vi "camera test.vi"() -> ()   [LabVIEW 2023]
uses:
  <vilib>/DAQmx/create/channels.llb/DAQmx Create Channel (DO-Digital Output).vi
  <vilib>/DAQmx/configure/timing.llb/DAQmx Timing (Sample Clock).vi
  <vilib>/Analysis/NI_AALBase.lvlib
  <vilib>/DAQmx/write.llb/DAQmx Write (Digital 1D U32 1Chan NSamp).vi
panel:
  in  "task in":refnum<k21>
  in  "low time":dbl=0.01 format="%.6f"
  in  "high time":dbl=0.01 format="%.6f"
  in  "OK Button":bool
  out "Pulse Pattern":dbl[](array[numeric])
  in  "source":tag
  in  "lines 2":tag
  in  "lines":tag
  in  "Advanced Genicam::Command Timeout":u32=100 max=0
  in  "Stop (F)":bool
  out "Image Out 2":T1(plugin-control)
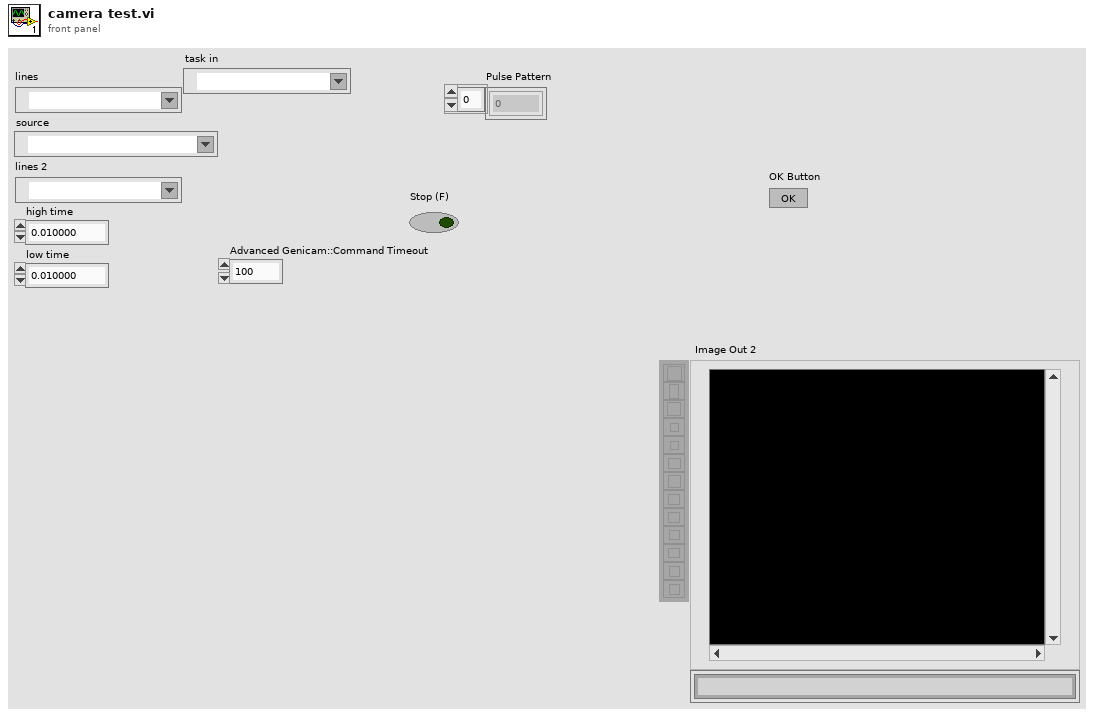
[diagram p1: front panel]
types:
  T1 = typedef "IMAQ Image.ctl" = refnum<image>
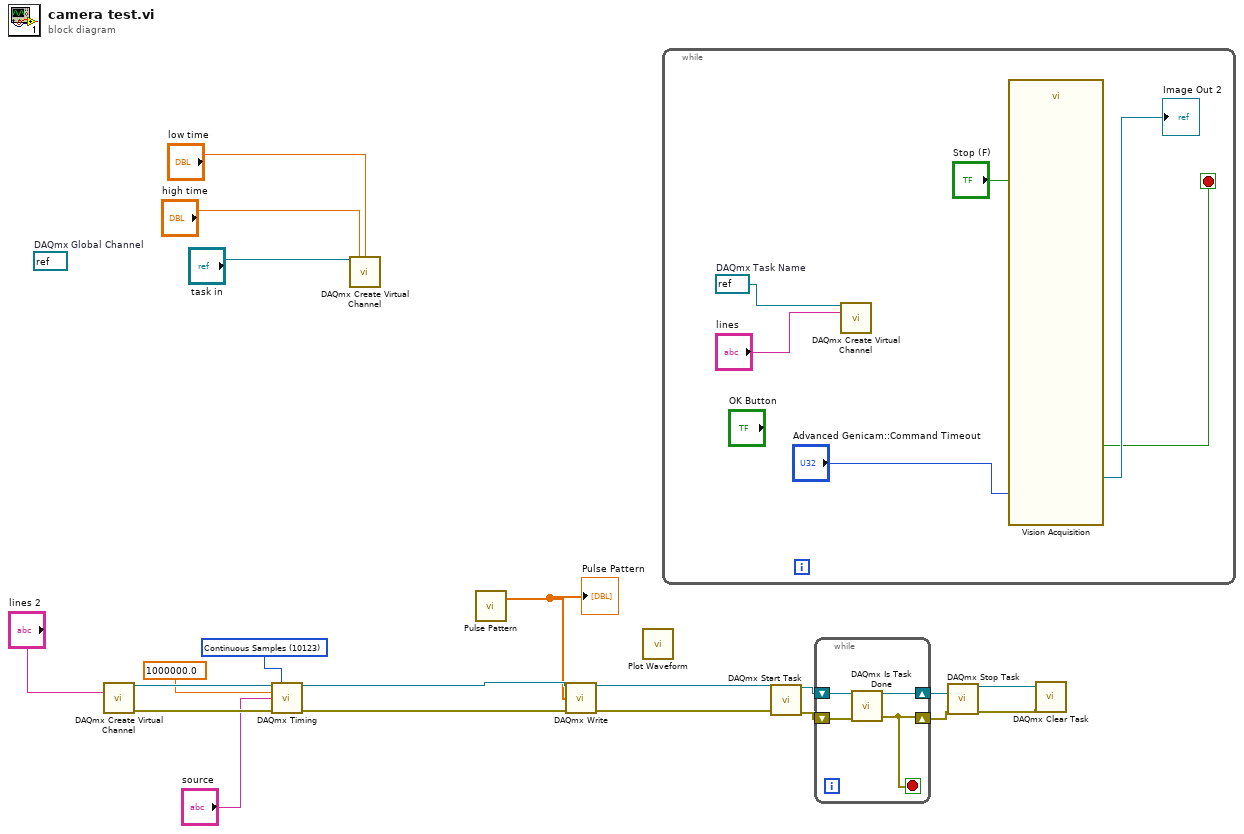
[diagram p0: block diagram]
diagram:
  (unwired) refnum<k21> refnum  # DAQmx Global Channel
  w15 = 10123 items=["Finite Samples"=10178, "Continuous Samples"=10123, "Hardware Timed Single Point"=12522] ("sample mode")
  n1 = call-poly <vilib>:"DAQmx Create Virtual Channel.vi"("lines"="lines 2") -> ("task out"=w19:refnum<k21>, "error out"=w18:errorcluster)  [unwired: 13 in]
  n2 = call-poly <vilib>:"DAQmx Timing.vi"("task/channels in"=w19, "sample mode"=w15, "rate"=1000000.0, "source"="source", "error in"=w18) -> ("task out"=w12:refnum<k21>, "error out"=w11:errorcluster)  [unwired: 9 in]
  n3 = call-poly <vilib>:"DAQmx Create Virtual Channel.vi"("task in"="task in", 1:"high time", 2:"low time") -> ()  [unwired: 11 in, 2 out]
  n4 = call <vilib>:"Pulse Pattern.vi"() -> ("Pulse Pattern"=w10:dbl[])  [unwired: 4 in, 1 out]
  "Pulse Pattern" <- w10
  n5 = call-poly <vilib>:"DAQmx Write.vi"("task/channels in"=w12, "data"=w10, "error in"=w11) -> ("task out"=w14:refnum<k21>, "error out"=w13:errorcluster)  [unwired: 10 in, 1 out]
  n6 = call <vilib>:"Plot Waveform.vi"() -> ()  [unwired: 11 in, 1 out]
  n7 = while {
    stop <- w24 stop-if-true
    w21 = refnum<k21> refnum  # DAQmx Task Name
    n8 = call-poly <vilib>:"DAQmx Create Virtual Channel.vi"("task in"=w21, "lines"="lines") -> ()  [unwired: 12 in, 2 out]
    n9 = call "Vision Acquisition"("Stop (F)"="Stop (F)", "Advanced Genicam::Command Timeout"="Advanced Genicam::Command Timeout") -> ("Image Out"=→"Image Out 2":T1, "Stopped"=w24:bool)  [unwired: 18 in, 6 out]
  }
  n10 = call <vilib>:"DAQmx Start Task.vi"("task/channels in"=w14, "error in"=w13) -> ("task out"=w9:refnum<k21>, "error out"=w8:errorcluster)  [unwired: 12 in]
  n11 = while {
    shift-right: [w28] -> w7
    shift-left: w9 -> [w30]
    shift-right: [w27] -> w6
    shift-left: w8 -> [w29]
    stop <- w27 stop-if-true
    n12 = call <vilib>:"DAQmx Is Task Done.vi"("task/channels in"=w30, "error in"=w29) -> ("task out"=w28:refnum<k21>, "error out"=w27:errorcluster)  [unwired: 11 in, 1 out]
  }
  n13 = call <vilib>:"DAQmx Stop Task.vi"("task/channels in"=w7, "error in"=w6) -> ("task out"=w5:refnum<k21>, "error out"=w4:errorcluster)  [unwired: 12 in]
  n14 = call <vilib>:"DAQmx Clear Task.vi"("task in"=w5, "error in"=w4) -> ()  [unwired: 13 in, 1 out]
